vi "Gunsim Precalc.vi"(3 "Robot Constants":T2={"Distance from Pivot Point to Drive Mount(in)"=2.0, "Distance from Pivot Point to Arm Mount(in)"=2.0, "Distance from Pivot Point to Launcher(in)"=2.0, "Distance from Pivot Point to Camera(in)"=2.0, "WheelEncoder Ticks/Revolution"=2.0, "Wheel Radius"=2.0, "Triangle Angle(degrees)"=2.0, "Minimum LA Distance(inches)"=2.0, "LA Distance/Tick(inches)"=2.0}, 4 "Framerate":i32, 5 "Other Constants":T3, 6 "Initial Velocity(in/s)":dbl) -> (0 "output cluster":T1, 1 "Wheel Power(ticks/100ms)":dbl, 2 "RPM":dbl)   [LabVIEW 2015]
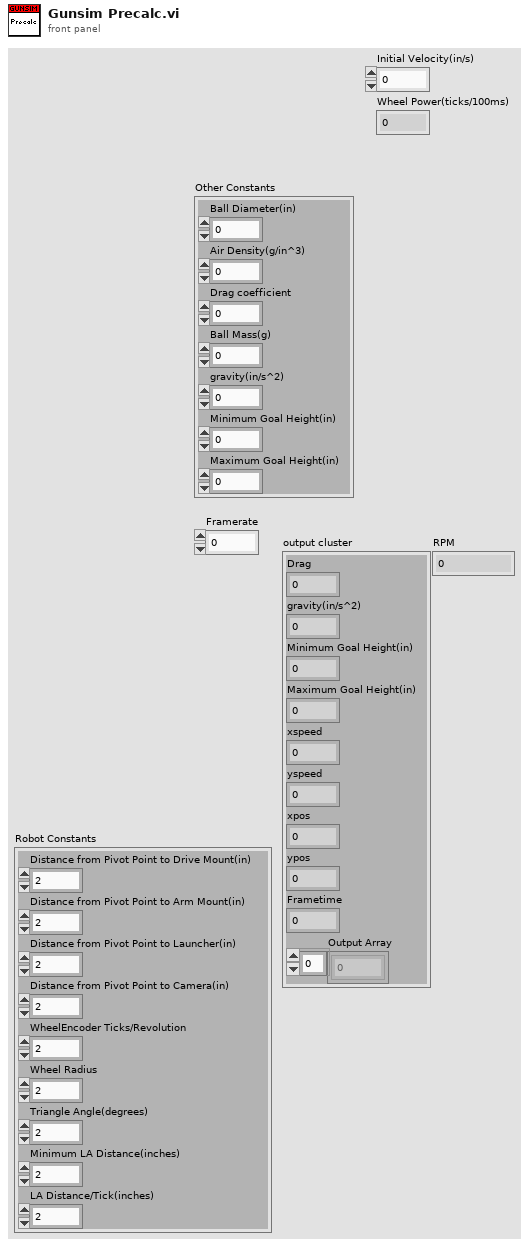
[diagram p1: front panel]
types:
  T1 = cluster{"Drag":dbl, "gravity(in/s^2)":dbl, "Minimum Goal Height(in)":dbl, "Maximum Goal Height(in)":dbl, "xspeed":dbl, "yspeed":dbl, "xpos":dbl, "ypos":dbl, "Frametime":dbl, "Output Array":dbl[]}
  T2 = cluster{"Distance from Pivot Point to Drive Mount(in)":dbl, "Distance from Pivot Point to Arm Mount(in)":dbl, "Distance from Pivot Point to Launcher(in)":dbl, "Distance from Pivot Point to Camera(in)":dbl, "WheelEncoder Ticks/Revolution":dbl, "Wheel Radius":dbl, "Triangle Angle(degrees)":dbl, "Minimum LA Distance(inches)":dbl, "LA Distance/Tick(inches)":dbl}
  T3 = cluster{"Ball Diameter(in)":dbl, "Air Density(g/in^3)":dbl, "Drag coefficient":dbl, "Ball Mass(g)":dbl, "gravity(in/s^2)":dbl, "Minimum Goal Height(in)":dbl, "Maximum Goal Height(in)":dbl}
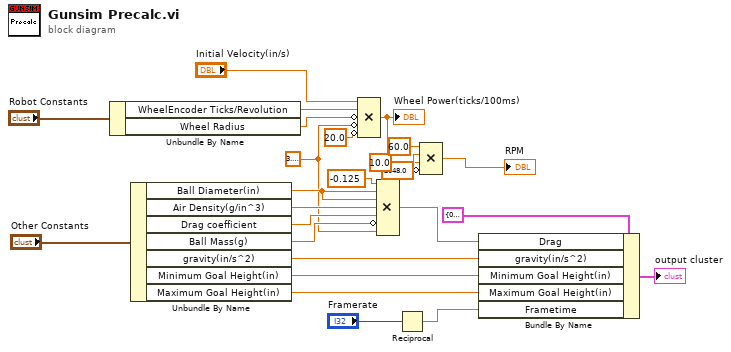
[diagram p0: block diagram]
diagram:
  w10 = 3.141592653589793
  n1 = Unbundle By Name("Robot Constants") -> ("WheelEncoder Ticks/Revolution"=w9:dbl, "Wheel Radius"=w8:dbl)
  n2 = Unbundle By Name("Other Constants") -> ("Ball Diameter(in)"=w15:dbl, "Air Density(g/in^3)"=w16:dbl, "Drag coefficient"=w17:dbl, "Ball Mass(g)"=w18:dbl, "gravity(in/s^2)"=w21:dbl, "Minimum Goal Height(in)"=w22:dbl, "Maximum Goal Height(in)"=w23:dbl)
  n3 = Compound Arithmetic op=MULTIPLY("Initial Velocity(in/s)", w9, invert w8, invert w10, invert 20.0 ("value")) -> (w3:dbl)
  "Wheel Power(ticks/100ms)" <- w3
  n4 = Compound Arithmetic op=MULTIPLY(-0.125 ("value"), w15, w15, w16, w17, invert w18, w10) -> (w19:dbl)
  n5 = Reciprocal(x="Framerate") -> (1/x=w25:dbl)
  n6 = Compound Arithmetic op=MULTIPLY(60.0 ("value"), w3, 10.0 ("value"), invert 2048.0 ("value")) -> (→"RPM":dbl)
  n7 = Bundle By Name(cluster=T1 {"Drag"=0.0, "gravity(in/s^2)"=-386.09, "Minimum Goal Height(in)"=85.0, "Maximum Goal Height(in)"=109.0, "xspeed"=0.0, "yspeed"=0.0, "xpos"=0.0, "ypos"=0.0, "Frametime"=0.0, "Output Array"=[]}, "Drag"=w19, "gravity(in/s^2)"=w21, "Minimum Goal Height(in)"=w22, "Maximum Goal Height(in)"=w23, "Frametime"=w25) -> (→"output cluster":T1)
